vi "BreakNemaIntoRecordsPerPoint.vi"(7 "elements":string[](array[string]), 8 "IpStatus (in)":T2[](array[typedef]) {"TimePing" scale=0.0..60.0; "%rtk" scale=0.0..60.0}, 11 "IP list":T1) -> (0 "IpStatus (out)":T2[](array[typedef]) {"TimePing" scale=0.0..60.0; "%rtk" scale=0.0..60.0}, 3 "IP list (out)":T1)   [LabVIEW 2012]
uses:
  GPS String Capture Software/IP RTK status Indicator.ctl
  ArrayIpAddressesAndReportingCheckbox.ctl
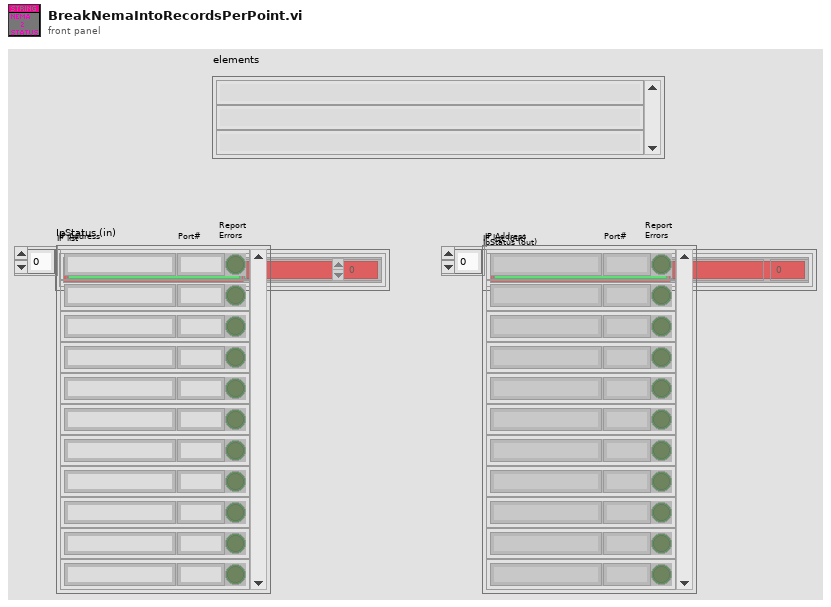
[diagram p1: front panel]
types:
  T1 = typedef "ArrayIpAddressesAndReportingCheckbox.ctl" = cluster{"IpAddress":string, "Report Errors":bool, "Port":string}[]
  T2 = typedef "IP RTK status Indicator.ctl" = cluster{"RTK Count":bool[], "Last Nema Time":dbl, "Last RTK Time":dbl, "Last Ping time":dbl, "Lastrtk":string, "IP":string, "TimePing":dbl, "%rtk":dbl, "MinLastRTk":dbl}
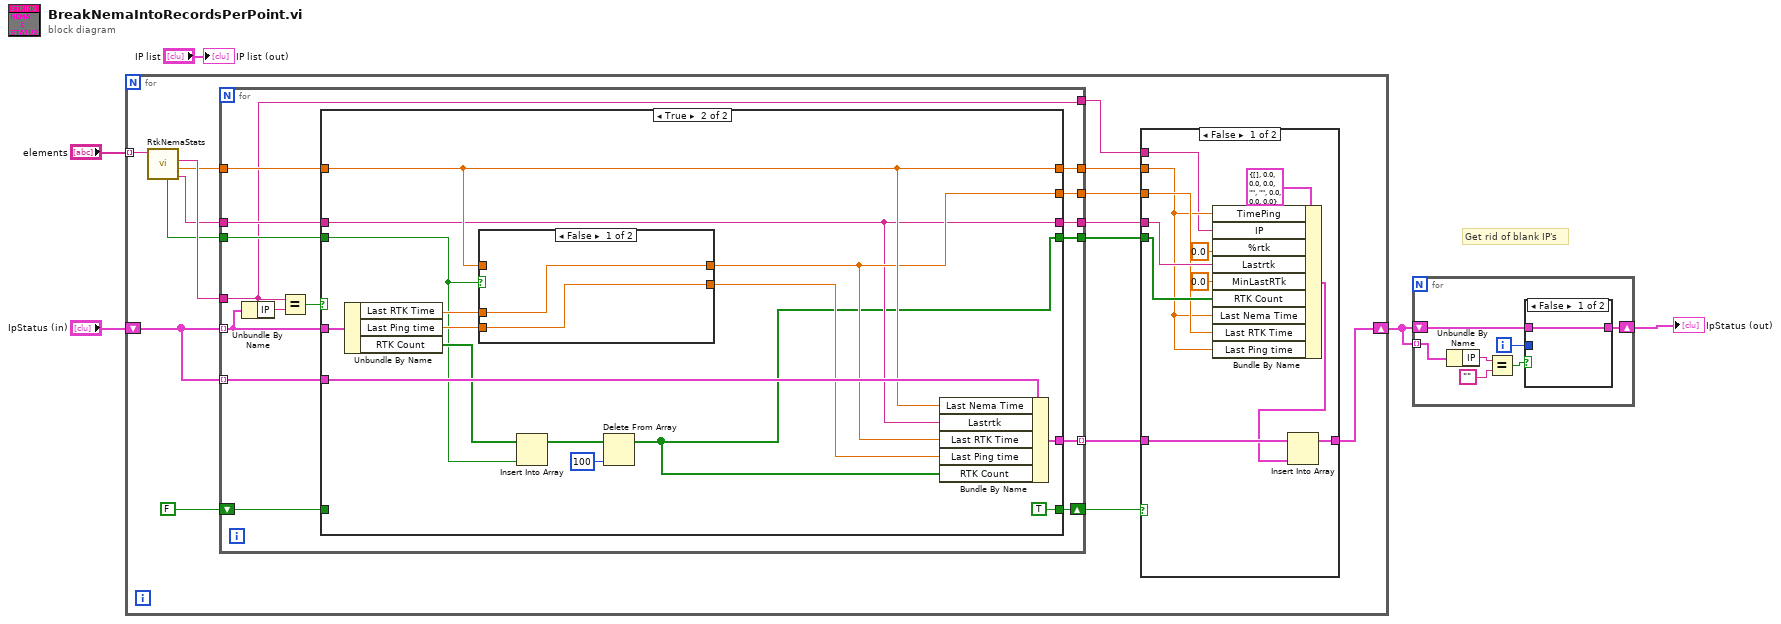
[diagram p0: block diagram]
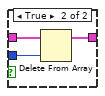
[diagram p2: hidden frame]
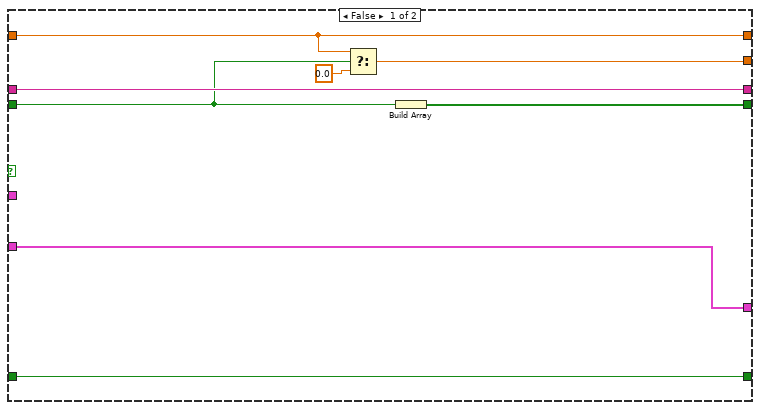
[diagram p4: hidden frame]
diagram:
  # "Get rid of blank IP's"
  n1 = for {
    tunnel: "elements" -> [w10] mode=indexing
    shift-right: [w17] -> w2
    shift-left: "IpStatus (in)" -> [w20]
    n2 = call "RtkNemaStats.vi"("Element"=w10) -> ("GPS Type"=w7:string, "Numeric Time Stamp"=w8:dbl, "IP-Port"=w9:string, "RTK = T"=w6:bool)  [unwired: 6 in, 1 out]
    n3 = for {
      tunnel: w20 -> [w40] mode=indexing
      tunnel: [w46] -> w16 mode=indexing
      tunnel: w9 -> [w33]
      tunnel: w6 -> [w43]
      tunnel: w7 -> [w42]
      tunnel: w20 -> [w41] mode=indexing
      shift-right: [w38] -> w18
      shift-left: FALSE -> [w39]
      tunnel: [w36] -> w14
      tunnel: [w35] -> w13
      tunnel: [w34] -> w12
      tunnel: [w33] -> w11
      tunnel: w8 -> [w47]
      tunnel: [w37] -> w15
      n4 = Unbundle By Name(w40) -> ("IP"=w45:string)
      n5 = Equal?(x=w33, y=w45) -> (x = y?=w44:bool)
      n6 = case shown="True" w44 {
        tunnel: w47 -> [w50 w59]
        tunnel: [w55 w70] -> w46
        tunnel: w43 -> [w51 w63]
        tunnel: w42 -> [w53 w57]
        tunnel: w41 -> [w55 w69]
        tunnel: w40 -> [_ w68]
        tunnel: w39 -> [w54 _]
        tunnel: [w54 TRUE] -> w38
        tunnel: [w50 w59] -> w37
        tunnel: [w53 w57] -> w36
        tunnel: [w52 w56] -> w35
        tunnel: [w48 w58] -> w34
        frame False {
          n7 = Select(t=w50, s=w51, f=0.0) -> (s? t:f=w48:dbl)
          n8 = Build Array(w51) -> (w52:bool[])
        }
        frame True {
          n9 = Unbundle By Name(w68) -> ("Last RTK Time"=w67:dbl, "Last Ping time"=w65:dbl, "RTK Count"=w64:bool[])
          n10 = case shown="False" w63 {
            tunnel: w67 -> [w72 _]
            tunnel: w59 -> [_ w73]
            tunnel: [w72 w73] -> w58
            tunnel: [w71 w73] -> w66
            tunnel: w65 -> [w71 _]
            frame False {
            }
            frame True {
            }
          }
          n11 = Insert Into Array(array=w64, new element=w63) -> (w62:bool[])  [unwired: 1 in]
          n12 = Delete From Array(array=w62, index=100) -> (array with subset deleted=w56:bool[])  [unwired: 1 in, 1 out]
          n13 = Bundle By Name(cluster=w69, "Last Nema Time"=w59, "Lastrtk"=w57, "Last RTK Time"=w58, "Last Ping time"=w66, "RTK Count"=w56) -> (w70:T2)
        }
      }
    }
    n14 = case shown="False" w18 {
      tunnel: [w30 w32] -> w17
      tunnel: w16 -> [w31 w32]
      tunnel: w15 -> [w24 _]
      tunnel: w14 -> [w27 _]
      tunnel: w13 -> [w26 _]
      tunnel: w12 -> [w25 _]
      tunnel: w11 -> [w23 _]
      frame False {
        n15 = Bundle By Name(cluster=T2 {"RTK Count"=[], "Last Nema Time"=0.0, "Last RTK Time"=0.0, "Last Ping time"=0.0, "Lastrtk"="", "IP"="", "TimePing"=0.0, "%rtk"=0.0, "MinLastRTk"=0.0} ("IP Status"), "TimePing"=w24, "IP"=w23, "%rtk"=0.0, "Lastrtk"=w27, "MinLastRTk"=0.0, "RTK Count"=w26, "Last Nema Time"=w24, "Last RTK Time"=w25, "Last Ping time"=w24) -> (w28:T2)
        n16 = Insert Into Array(array=w31, new element=w28) -> (w30:T2[])  [unwired: 1 in]
      }
      frame True {
      }
    }
  }
  n17 = for {
    tunnel: w2 -> [w77] mode=indexing
    shift-right: [w75] -> w1
    shift-left: w2 -> [w76]
    i -> [w74]
    n18 = Unbundle By Name(w77) -> ("IP"=w80:string)
    n19 = Equal?(x=w80, y="") -> (x = y?=w78:bool)
    n20 = case shown="False" w78 {
      tunnel: w76 -> [w81 w84]
      tunnel: [w81 w83] -> w75
      tunnel: w74 -> [_ w82]
      frame False {
      }
      frame True {
        n21 = Delete From Array(array=w84, index=w82) -> (array with subset deleted=w83:T2[])  [unwired: 1 in, 1 out]
      }
    }
  }
  "IpStatus (out)" <- w1
  "IP list (out)" <- "IP list"
